vi "Count Coins - Video.vi"() -> ()   [LabVIEW 2025]
uses:
  <vilib>/vision/driver/NI_Vision_Acquisition_Software.lvlib
  <vilib>/userDefined/High Color/IMAQdx.ctl
  Coin Analyser/Coin Analyser.lvclass
  <vilib>/vision/driver/IMAQdx.llb/IMAQdx Camera Control Mode.ctl
  <vilib>/Python/Open Venv Python Session.vi
panel:
  out "Coins":i32
  out "Processed fps":dbl
  out "Coins":cluster{"x":i32, "y":i32, "diameter":i32}[](array[cluster])
  in  "stop":bool
  out "Image":T1(plugin-control)
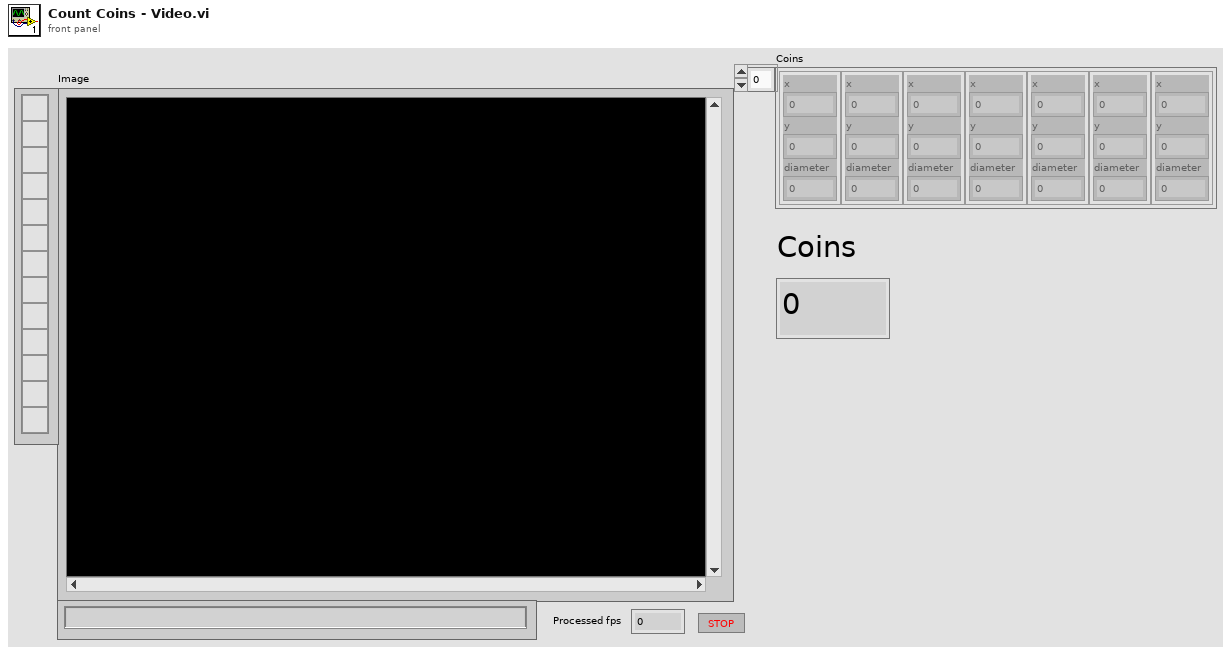
[diagram p1: front panel]
types:
  T1 = typedef "IMAQ Image.ctl" = refnum<image>
  T2 = typedef "NI_Vision_Acquisition_Software.lvlib/IMAQdx Camera Control Mode.ctl" = enum32{"Controller", "Listener"}
  T3 = typedef "IMAQdx.ctl" = refnum<k21>
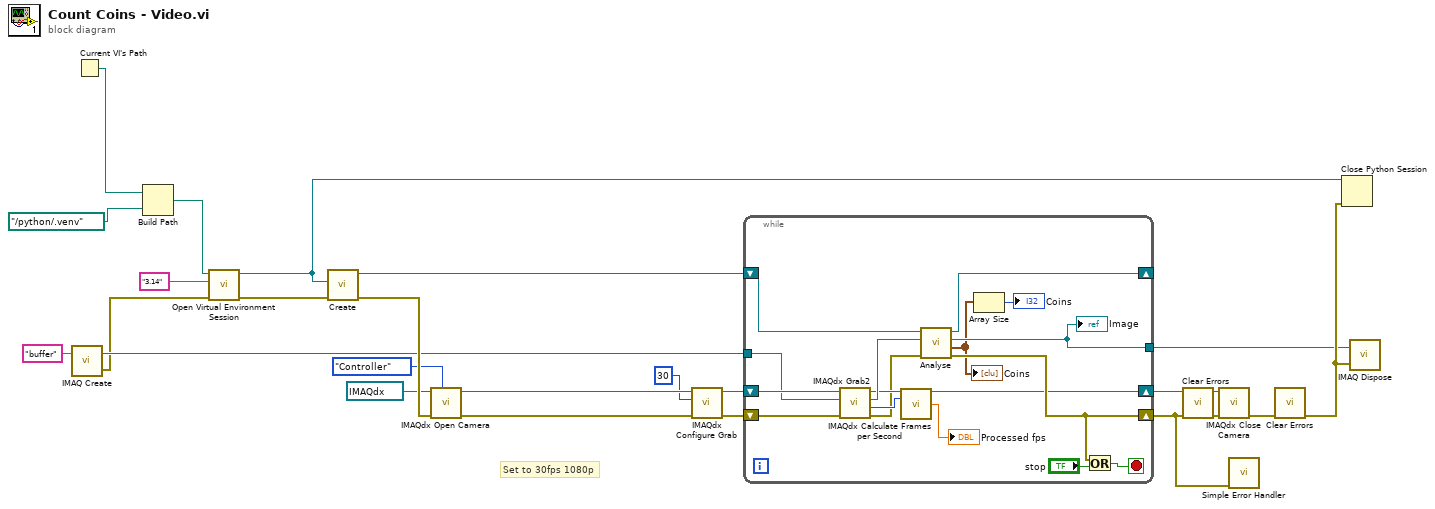
[diagram p0: block diagram]
diagram:
  # "Set to 30fps 1080p"
  n1 = call "IMAQ Create"("Image Name"="buffer") -> ("New Image"=w18:T1, "error out"=w7:errorcluster)  [unwired: 4 in]
  n2 = Current VI's Path() -> (path=w3:path)
  n3 = Build Path(base path=w3, name or relative path=path "../python/.venv" ("Env path")) -> (appended path=w1:path)
  n4 = call-poly <vilib>:"Open Virtual Environment Session.vi"("error in (no error)"=w7, "Python version"="3.14", "Env path"=w1) -> ("error out"=w5:errorcluster, "session out"=w4:refnum<k35>)  [unwired: 7 in]
  n5 = call "Create.vi"("error in (no error)"=w5, "session"=w4) -> ("error out"=w23:errorcluster, "Coin Analyser out"=w22:refnum<class "Coin Analyser.lvclass">)  [unwired: 8 in]
  n6 = call <vilib>:"IMAQdx Open Camera.vi"("Camera Control Mode"=IMAQdx_Camera_Control_Mode."Controller", "error in"=w23, "Session In"=T3 "cam0") -> ("error out"=w12:errorcluster, "Session Out"=w13:T3)  [unwired: 7 in]
  n7 = call <vilib>:"IMAQdx Configure Grab.vi"("error in"=w12, "Number of Buffers"=u32 30, "Session In"=w13) -> ("error out"=w19:errorcluster, "Session Out"=w20:T3)  [unwired: 7 in]
  n8 = while {
    tunnel: w18 -> [w38]
    shift-right: [w31] -> w17
    shift-left: w20 -> [w40]
    shift-right: [w34] -> w15
    shift-left: w19 -> [w39]
    shift-right: [w33] -> _
    shift-left: w22 -> [w41]
    tunnel: [w28] -> w10
    stop <- w35 stop-if-true
    n9 = call <vilib>:"IMAQdx Grab2.vi"("error in"=w39, "Image In"=w38, "Session In"=w40) -> ("error out"=w27:errorcluster, "Buffer Number Out"=w30:u32, "Image Out"=w37:T1, "Session Out"=w32:T3)  [unwired: 5 in]
    n10 = call <vilib>:"IMAQdx Calculate Frames per Second.vi"("Session In"=w32, "Buffer Number"=w30) -> ("Session Out"=w31:T3, "Processed Frames per Second"=→"Processed fps":dbl)  [unwired: 7 in, 5 out]
    n11 = call "Analyse.vi"("error in (no error)"=w27, "Image in"=w37, "Coin Analyser in"=w41) -> ("error out"=w34:errorcluster, "Coins"=w26:cluster{"x":i32, "y":i32, "diameter":i32}[], "Image Out"=w28:T1, "Coin Analyser out"=w33:refnum<class "Coin Analyser.lvclass">)  [unwired: 5 in]
    "Image" <- w28
    "Coins" <- w26
    n12 = Array Size(array=w26) -> (size(s)=→"Coins":i32)
    n13 = Or(x=w34, y="stop") -> (x .or. y?=w35:bool)
  }
  n14 = call <vilib>:"Clear Errors.vi"("error in (no error)"=w15) -> ("error out"=w14:errorcluster)  [unwired: 5 in, 1 out]
  n15 = call <vilib>:"IMAQdx Close Camera.vi"("error in"=w14, "Session In"=w17) -> ("error out"=w16:errorcluster)  [unwired: 9 in]
  n16 = call <vilib>:"Simple Error Handler.vi"("error in (no error)"=w15) -> ()  [unwired: 4 in, 5 out]
  n17 = call <vilib>:"Clear Errors.vi"("error in (no error)"=w16) -> ("error out"=w11:errorcluster)  [unwired: 5 in, 1 out]
  n18 = Close Python Session(session in=w4, error in=w11) -> ()  [unwired: 1 out]
  n19 = call "IMAQ Dispose"("Image"=w10, "error in (no error)"=w11) -> ()  [unwired: 4 in, 1 out]
